vi "Walk through Variant recursive.vi"(8 "error in":errorcluster, 9 "Section":string, 10 "Type in":variant, 11 "Node in":variant) -> (0 "error out":errorcluster, 3 "Node out":variant)   [LabVIEW 2022 SP3, in "hse-config.lvlib" / "config-base.lvclass"]
doc: "____\nHAMPEL SOFTWARE ENGINEERING v3.8.0 (2023-12-18 14:41)"
uses:
  config-base.lvclass
  hse-misc/Type_Descriptor/TypeDescriptor_GetPString.vi
  hse-misc/Conversion/Variant_EmptyCluster.vi
  <vilib>/Utility/GetType.llb/TD_Create Cluster.vi
  <vilib>/Utility/Data Type/NI_Data Type.lvlib
  hse-misc/hse-misc.lvlib
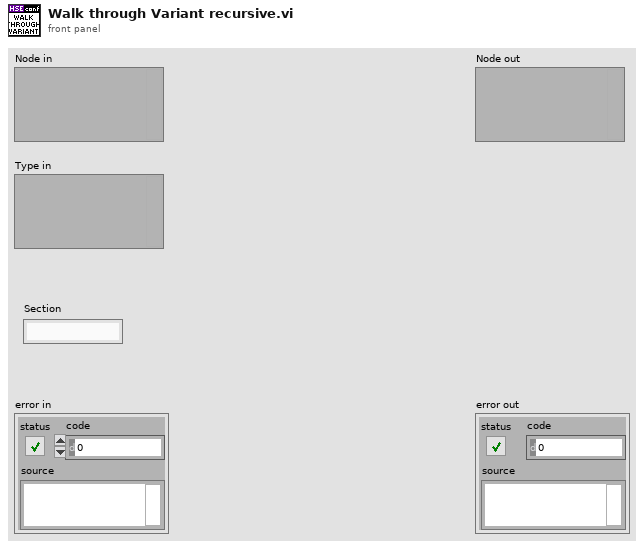
[diagram p1: front panel]
types:
  T1 = typedef "NI_Data Type.lvlib/Data Type.ctl" = enum8{"Invalid Type", "Void", "I8", "I16", "I32", "I64", "U8", "U16", "U32", "U64", "Single Float", "Double Float", "Extended Float", "Single Complex", "Double Complex", "Extended Complex", "Enum U8", "Enum U16", "Enum U32", "Enum U64", "Single Float With Unit", "Double Float With Unit", "Extended Float With Unit", "Single Complex with Unit", "Double Complex with Unit", "Extended Complex with Unit", "Boolean", "String", "Path", "Picture", "Tag", "Array", "Cluster", "Variant", "LV Variant", "Waveform", "Timestamp", "Digital Waveform", "Digital Data", "ExpressData", "Refnum", "External Data", "VI", "Poly VI", "LabVIEW Class Instance", "Fixed Point", "Set Collection", "Map Collection"}
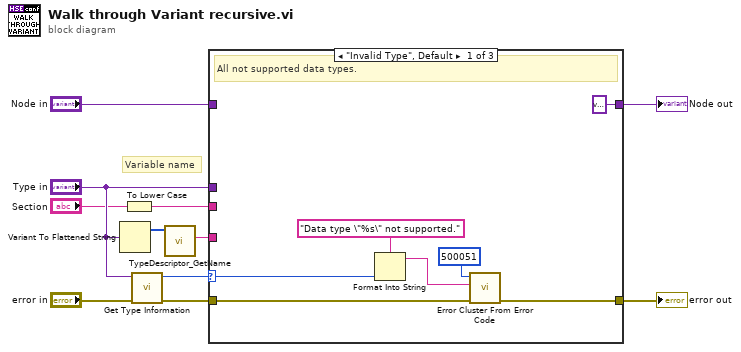
[diagram p0: block diagram]
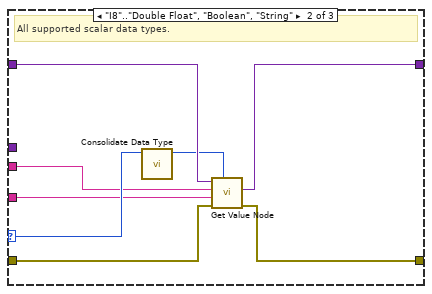
[diagram p2: hidden frame]
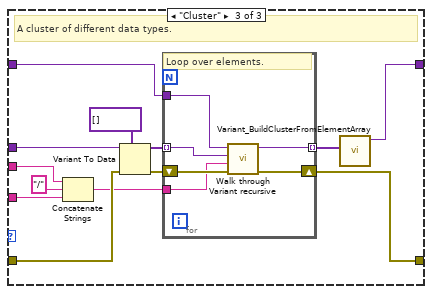
[diagram p3: hidden frame]
diagram:
  # "Variable name"
  n1 = Variant To Flattened String(Variant="Type in") -> (1:w6:i16[])  [unwired: 1 out]
  n2 = To Lower Case(string="Section") -> (all lower case string=w1:string)
  n3 = call <vilib>:"Get Type Information.vi"("error in (no error)"="error in", "variant"="Type in") -> ("error out"=w5:errorcluster, "type"=w4:T1)  [unwired: 5 in, 3 out]
  n4 = call "TypeDescriptor_GetName.vi"("type descriptor"=w6) -> ("name"=w8:string)  [unwired: 8 in, 2 out]
  n5 = case shown="\"Invalid Type\", Default" w4 {
    selector: w4 -> [w13 w24 _]
    tunnel: w5 -> [w15 w25 w38]
    tunnel: "Type in" -> [_ _ w39]
    tunnel: [w14 w21 w31] -> w10
    tunnel: w8 -> [_ w20 w29]
    tunnel: "Node in" -> [_ w26 w34]
    tunnel: [variant ("Root Node") w22 w32] -> w11
    tunnel: w1 -> [_ w19 w30]
    frame "Invalid Type", Default {
      # "All not supported data types."
      n6 = Format Into String(format string="Data type \"%s\" not supported.", w13) -> (resulting string=w17:string)  [unwired: 2 in, 1 out]
      n7 = call <vilib>:"Error Cluster From Error Code.vi"("error in (no error)"=w15, "error message (\"\")"=w17, "error code (0)"=500051) -> ("error out"=w14:errorcluster)  [unwired: 6 in]
    }
    frame "I8".."Double Float", "Boolean", "String" {
      # "All supported scalar data types."
      n8 = call "Consolidate Data Type.vi"("Type in"=w24) -> ("Type out"=w23:T1)  [unwired: 10 in]
      n9 = call "Get Value Node.vi"("Data Type"=w23, "error in"=w25, "Key"=w20, "Section"=w19, "Root Node"=w26) -> ("error out"=w21:errorcluster, "Value Node out"=w22:variant)  [unwired: 5 in]
    }
    frame "Cluster" {
      # "A cluster of different data types."
      n10 = Concatenate Strings(w30, "/" ("element"), w29) -> (w28:string)
      n11 = Variant To Data(error in=w38, type=variant[] [], Variant=w39) -> (data=w36:variant[], error out=w35:errorcluster)
      n12 = for {
        tunnel: w36 -> [w42] mode=indexing
        shift-right: [w41] -> w31
        shift-left: w35 -> [w45]
        tunnel: [w44] -> w33 mode=indexing
        tunnel: w34 -> [w43]
        tunnel: w28 -> [w40]
        # "Loop over elements."
        n13 = call "Walk through Variant recursive.vi"("error in"=w45, "Section"=w40, "Type in"=w42, "Node in"=w43) -> ("error out"=w41:errorcluster, "Node out"=w44:variant)  [unwired: 6 in]
      }
      n14 = call "Variant_BuildClusterFromElementArray.vi"("Elements"=w33) -> ("Cluster"=w32:variant)  [unwired: 10 in]
    }
  }
  "Node out" <- w11
  "error out" <- w10
